vi "main.vi"() -> ()   [LabVIEW 2023] (continued)
20\tFF\tFF\tFF\tFF\tFF\tFF\r\n       952  1FFFFFFF   00000004    8        00\t00\tFF\tFF\tFF\tFF\tFF\tFF\r\n       947  1FFFFFFF   00000004    8        00\t00\tFF\tFF\tFF\tFF\tFF\tFF\r\n       946  18F121F0   00000004    8        09\t16\t00\t00\tFF\tFF\tB0\t01\r\n       993  18F106A7   00000004    8        00\tF7\tFF\tFF\tFF\tFF\tFF\t84\r\n       992  1FFFFFFF   00000004    8        00\t00\tFF\tFF\tFF\tFF\tFF\tFF\r\n       983  0CF102A7   00000004    8        30\t75\tE0\t2E\t80\tFF\tFF\tFD\r\n       983  0CF101A7   00000004    8        68\t00\t97\tCC\t00\t15\t39\t4B\r\n       982  1FFFFFFF   00000004    8        00\t00\tFF\tFF\tFF\tFF\tFF\tFF\r\n       972  1FFFFFFF   00000004    8        00\t00\tFF\tFF\tFF\tFF\tFF\tFF\r\n       963  0CF102A7   00000004    8        30\t75\tE0\t2E\t80\tFF\tFF\tFD\r\n       963  0CF101A7   00000004    8        68\t00\t97\tCC\t00\t15\t39\t4A\r\n       962  1FFFFFFF   00000004    8        00\t20\tFF\tFF\tFF\tFF\tFF\tFF\r\n       952  1FFFFFFF   00000004    8        00\t00\tFF\tFF\tFF\tFF\tFF\tFF\r\n       947  1FFFFFFF   00000004    8        00\t00\tFF\tFF\tFF\tFF\tFF\tFF\r\n      1002  1FFFFFFF   00000004    8        00\t00\tFF\tFF\tFF\tFF\tFF\tFF\r\n       993  18F106A7   00000004    8        00\tF7\tFF\tFF\tFF\tFF\tFF\t84\r\n       992  1FFFFFFF   00000004    8        00\t00\tFF\tFF\tFF\tFF\tFF\tFF\r\n       983  0CF102A7   00000004    8        30\t75\tE0\t2E\t80\tFF\tFF\tFD\r\n       983  0CF101A7   00000004    8        68\t00\t97\tCC\t00\t15\t39\t4B\r\n       982  1FFFFFFF   00000004    8        00\t00\tFF\tFF\tFF\tFF\tFF\tFF\r\n       972  1FFFFFFF   00000004    8        00\t00\tFF\tFF\tFF\tFF\tFF\tFF\r\n       963  0CF102A7   00000004    8        30\t75\tE0\t2E\t80\tFF\tFF\tFD\r\n       963  0CF101A7   00000004    8        68\t00\t97\tCC\t00\t15\t39\t4A\r\n       962  1FFFFFFF   00000004    8        00\t20\tFF\tFF\tFF\tFF\tFF\tFF\r\n       952  1FFFFFFF   00000004    8        00\t00\tFF\tFF\tFF\tFF\tFF\tFF\r\n      1003  0CF101A7   00000004    8        68\t00\t97\tCC\t00\t15\t39\t4C\r\n      1002  1FFFFFFF   00000004    8        00\t00\tFF\tFF\tFF\tFF\tFF\tFF\r\n       993  18F106A7   00000004    8        00\tF7\tFF\tFF\tFF\tFF\tFF\t84\r\n       992  1FFFFFFF   00000004    8        00\t00\tFF\tFF\tFF\tFF\tFF\tFF\r\n       983  0CF102A7   00000004    8        30\t75\tE0\t2E\t80\tFF\tFF\tFD\r\n       983  0CF101A7   00000004    8        68\t00\t97\tCC\t00\t15\t39\t4B\r\n       982  1FFFFFFF   00000004    8        00\t00\tFF\tFF\tFF\tFF\tFF\tFF\r\n       972  1FFFFFFF   00000004    8        00\t00\tFF\tFF\tFF\tFF\tFF\tFF\r\n       963  0CF102A7   00000004    8        30\t75\tE0\t2E\t80\tFF\tFF\tFD\r\n       963  0CF101A7   00000004    8        68\t00\t97\tCC\t00\t15\t39\t4A\r\n       962  1FFFFFFF   00000004    8        00\t20\tFF\tFF\tFF\tFF\tFF\tFF\r\n      1003  0CF102A7   00000004    8        30\t75\tE0\t2E\t80\tFF\tFF\tFD\r\n      1003  0CF101A7   00000004    8        68\t00\t97\tCC\t00\t15\t39\t4C\r\n      1002  1FFFFFFF   00000004    8        00\t00\tFF\tFF\tFF\tFF\tFF\tFF\r\n       993  18F106A7   00000004    8        00\tF7\tFF\tFF\tFF\tFF\tFF\t84\r\n       992  1FFFFFFF   00000004    8        00\t00\tFF\tFF\tFF\tFF\tFF\tFF\r\n       983  0CF102A7   00000004    8        30\t75\tE0\t2E\t80\tFF\tFF\tFD\r\n       983  0CF101A7   00000004    8        68\t00\t97\tCC\t00\t15\t39\t4B\r\n       982  1FFFFFFF   00000004    8        00\t00\tFF\tFF\tFF\tFF\tFF\tFF\r\n       972  1FFFFFFF   00000004    8        00\t00\tFF\tFF\tFF\tFF\tFF\tFF\r\n       963  0CF102A7   00000004    8        30\t75\tE0\t2E\t80\tFF\tFF\tFD\r\n       963  0CF101A7   00000004    8        68\t00\t97\tCC\t00\t15\t39\t4A\r\n      1012  1FFFFFFF   00000004    8        00\t00\tFF\tFF\tFF\tFF\tFF\tFF\r\n      1003  0CF102A7   00000004    8        30\t75\tE0\t2E\t80\tFF\tFF\tFD\r\n      1003  0CF101A7   00000004    8        68\t00\t97\tCC\t00\t15\t39\t4C\r\n      1002  1FFFFFFF   00000004    8        00\t00\tFF\tFF\tFF\tFF\tFF\tFF\r\n       993  18F106A7   00000004    8        00\tF7\tFF\tFF\tFF\tFF\tFF\t84\r\n       992  1FFFFFFF   00000004    8        00\t00\tFF\tFF\tFF\tFF\tFF\tFF\r\n       983  0CF102A7   00000004    8        30\t75\tE0\t2E\t80\tFF\tFF\tFD\r\n       983  0CF101A7   00000004    8        68\t00\t97\tCC\t00\t15\t39\t4B\r\n       982  1FFFFFFF   00000004    8        00\t00\tFF\tFF\tFF\tFF\tFF\tFF\r\n       972  1FFFFFFF   00000004    8        00\t00\tFF\tFF\tFF\tFF\tFF\tFF\r\n       963  0CF102A7   00000004    8        30\t75\tE0\t2E\t80\tFF\tFF\tFD\r\n      1022  1FFFFFFF   00000004    8        00\t20\tFF\tFF\tFF\tFF\tFF\tFF\r\n      1012  1FFFFFFF   00000004    8        00\t00\tFF\tFF\tFF\tFF\tFF\tFF\r\n      1003  0CF102A7   00000004    8        30\t75\tE0\t2E\t80\tFF\tFF\tFD\r\n      1003  0CF101A7   00000004    8        68\t00\t97\tCC\t00\t15\t39\t4C\r\n      1002  1FFFFFFF   00000004    8        00\t00\tFF\tFF\tFF\tFF\tFF\tFF\r\n       993  18F106A7   00000004    8        00\tF7\tFF\tFF\tFF\tFF\tFF\t84\r\n       992  1FFFFFFF   00000004    8        00\t00\tFF\tFF\tFF\tFF\tFF\tFF\r\n       983  0CF102A7   00000004    8        30\t75\tE0\t2E\t80\tFF\tFF\tFD\r\n       983  0CF101A7   00000004    8        68\t00\t97\tCC\t00\t15\t39\t4B\r\n       982  1FFFFFFF   00000004    8        00\t00\tFF\tFF\tFF\tFF\tFF\tFF\r\n       972  1FFFFFFF   00000004    8        00\t00\tFF\tFF\tFF\tFF\tFF\tFF\r\n      1023  0CF101A7   00000004    8        68\t00\t97\tCC\t00\t15\t39\t4D\r\n      1022  1FFFFFFF   00000004    8        00\t20\tFF\tFF\tFF\tFF\tFF\tFF\r\n      1012  1FFFFFFF   00000004    8        00\t00\tFF\tFF\tFF\tFF\tFF\tFF\r\n      1003  0CF102A7   00000004    8        30\t75\tE0\t2E\t80\tFF\tFF\tFD\r\n      1003  0CF101A7   00000004    8        68\t00\t97\tCC\t00\t15\t39\t4C\r\n      1002  1FFFFFFF   00000004    8        00\t00\tFF\tFF\tFF\tFF\tFF\tFF\r\n       993  18F106A7   00000004    8        00\tF7\tFF\tFF\tFF\tFF\tFF\t84\r\n       992  1FFFFFFF   00000004    8        00\t00\tFF\tFF\tFF\tFF\tFF\tFF\r\n       983  0CF102A7   00000004    8        30\t75\tE0\t2E\t80\tFF\tFF\tFD\r\n       983  0CF101A7   00000004    8        68\t00\t97\tCC\t00\t15\t39\t4B\r\n       982  1FFFFFFF   00000004    8        00\t00\tFF\tFF\tFF\tFF\tFF\tFF\r\n      1023  0CF102A7   00000004    8        30\t75\tE0\t2E\t80\tFF\tFF\tFD\r\n      1023  0CF101A7   00000004    8        68\t00\t97\tCC\t00\t15\t39\t4D\r\n      1022  1FFFFFFF   00000004    8        00\t20\tFF\tFF\tFF\tFF\tFF\tFF\r\n      1012  1FFFFFFF   00000004    8        00\t00\tFF\tFF\tFF\tFF\tFF\tFF\r\n      1003  0CF102A7   00000004    8        30\t75\tE0\t2E\t80\tFF\tFF\tFD\r\n      1003  0CF101A7   00000004    8        68\t00\t97\tCC\t00\t15\t39\t4C\r\n      1002  1FFFFFFF   00000004    8        00\t00\tFF\tFF\tFF\tFF\tFF\tFF\r\n       993  18F106A7   00000004    8        00\tF7\tFF\tFF\tFF\tFF\tFF\t84\r\n       992  1FFFFFFF   00000004    8        00\t00\tFF\tFF\tFF\tFF\tFF\tFF\r\n       983  0CF102A7   00000004    8        30\t75\tE0\t2E\t80\tFF\tFF\tFD\r\n       983  0CF101A7   00000004    8        68\t00\t97\tCC\t00\t15\t39\t4B\r\n      1032  1FFFFFFF   00000004    8        00\t00\tFF\tFF\tFF\tFF\tFF\tFF\r\n      1023  0CF102A7   00000004    8        30\t75\tE0\t2E\t80\tFF\tFF\tFD\r\n      1023  0CF101A7   00000004    8        68\t00\t97\tCC\t00\t15\t39\t4D\r\n      1022  1FFFFFFF   00000004    8        00\t20\tFF\tFF\tFF\tFF\tFF\tFF\r\n      1012  1FFFFFFF   00000004    8        00\t00\tFF\tFF\tFF\tFF\tFF\tFF\r\n      1003  0CF102A7   00000004    8        30\t75\tE0\t2E\t80\tFF\tFF\tFD\r\n      1003  0CF101A7   00000004    8        68\t00\t97\tCC\t00\t15\t39\t4C\r\n      1002  1FFFFFFF   00000004    8        00\t00\tFF\tFF\tFF\tFF\tFF\tFF\r\n       993  18F106A7   00000004    8        00\tF7\tFF\tFF\tFF\tFF\tFF\t84\r\n       992  1FFFFFFF   00000004    8        00\t00\tFF\tFF\tFF\tFF\tFF\tFF\r\n       983  0CF102A7   00000004    8        30\t75\tE0\t2E\t80\tFF\tFF\tFD\r\n      1041  18F11FF0   00000004    8        FF\t3F\t90\t68\t88\t1B\t10\t2C\r\n      1032  1FFFFFFF   00000004    8        00\t00\tFF\tFF\tFF\tFF\tFF\tFF\r\n      1023  0CF102A7   00000004    8        30\t75\tE0\t2E\t80\tFF\tFF\tFD\r\n      1023  0CF101A7   00000004    8        68\t00\t97\tCC\t00\t15\t39\t4D\r\n      1022  1FFFFFFF   00000004    8        00\t20\tFF\tFF\tFF\tFF\tFF\tFF\r\n      1012  1FFFFFFF   00000004    8        00\t00\tFF\tFF\tFF\tFF\tFF\tFF\r\n      1003  0CF102A7   00000004    8        30\t75\tE0\t2E\t80\tFF\tFF\tFD\r\n      1003  0CF101A7   00000004    8        68\t00\t97\tCC\t00\t15\t39\t4C\r\n      1002  1FFFFFFF   00000004    8        00\t00\tFF\tFF\tFF\tFF\tFF\tFF\r\n       993  18F106A7   00000004    8        00\tF7\tFF\tFF\tFF\tFF\tFF\t84\r\n       992  1FFFFFFF   00000004    8        00\t00\tFF\tFF\tFF\tFF\tFF\tFF\r\n      1042  18F120F0   00000004    8        2B\t75\t60\tB1\tB0\t01\tFF\tFF\r\n      1041  18F11FF0   00000004    8        FF\t3F\t90\t68\t88\t1B\t10\t2C\r\n      1032  1FFFFFFF   00000004    8        00\t00\tFF\tFF\tFF\tFF\tFF\tFF\r\n      1023  0CF102A7   00000004    8        30\t75\tE0\t2E\t80\tFF\tFF\tFD\r\n      1023  0CF101A7   00000004    8        68\t00\t97\tCC\t00\t15\t39\t4D\r\n      1022  1FFFFFFF   00000004    8        00\t20\tFF\tFF\tFF\tFF\tFF\tFF\r\n      1012  1FFFFFFF   00000004    8        00\t00\tFF\tFF\tFF\tFF\tFF\tFF\r\n      1003  0CF102A7   00000004    8        30\t75\tE0\t2E\t80\tFF\tFF\tFD\r\n      1003  0CF101A7   00000004    8        68\t00\t97\tCC\t00\t15\t39\t4C\r\n      1002  1FFFFFFF   00000004    8        00\t00\tFF\tFF\tFF\tFF\tFF\tFF\r\n       993  18F106A7   00000004    8        00\tF7\tFF\tFF\tFF\tFF\tFF\t84\r\n      1043  0CF101A7   00000004    8        68\t00\t97\tCC\t00\t15\t39\t4E\r\n      1042  18F120F0   00000004    8        2B\t75\t60\tB1\tB0\t01\tFF\tFF\r\n      1041  18F11FF0   00000004    8        FF\t3F\t90\t68\t88\t1B\t10\t2C\r\n      1032  1FFFFFFF   00000004    8        00\t00\tFF\tFF\tFF\tFF\tFF\tFF\r\n      1023  0CF102A7   00000004    8        30\t75\tE0\t2E\t80\tFF\tFF\tFD\r\n      1023  0CF101A7   00000004    8        68\t00\t97\tCC\t00\t15\t39\t4D\r\n      1022  1FFFFFFF   00000004    8        00\t20\tFF\tFF\tFF\tFF\tFF\tFF\r\n      1012  1FFFFFFF   00000004    8        00\t00\tFF\tFF\tFF\tFF\tFF\tFF\r\n      1003  0CF102A7   00000004    8        30\t75\tE0\t2E\t80\tFF\tFF\tFD\r\n      1003  0CF101A7   00000004    8        68\t00\t97\tCC\t00\t15\t39\t4C\r\n      1002  1FFFFFFF   00000004    8        00\t00\tFF\tFF\tFF\tFF\tFF\tFF\r\n      1043  0C3C4D4A   00000004    8        BE\tFF\tFF\t7F\t18\tFF\tFF\t42\r\n      1043  0CF101A7   00000004    8        68\t00\t97\tCC\t00\t15\t39\t4E\r\n      1042  18F120F0   00000004    8        2B\t75\t60\tB1\tB0\t01\tFF\tFF\r\n      1041  18F11FF0   00000004    8        FF\t3F\t90\t68\t88\t1B\t10\t2C\r\n      1032  1FFFFFFF   00000004    8        00\t00\tFF\tFF\tFF\tFF\tFF\tFF\r\n      1023  0CF102A7   00000004    8        30\t75\tE0\t2E\t80\tFF\tFF\tFD\r\n      1023  0CF101A7   00000004    8        68\t00\t97\tCC\t00\t15\t39\t4D\r\n      1022  1FFFFFFF   00000004    8        00\t20\tFF\tFF\tFF\tFF\tFF\tFF\r\n      1012  1FFFFFFF   00000004    8        00\t00\tFF\tFF\tFF\tFF\tFF\tFF\r\n      1003  0CF102A7   00000004    8        30\t75\tE0\t2E\t80\tFF\tFF\tFD\r\n      1003  0CF101A7   00000004    8        68\t00\t97\tCC\t00\t15\t39\t4C\r\n      1044  0CF102A7   00000004    8        30\t75\tE0\t2E\t80\tFF\tFF\tFD\r\n      1043  0C3C4D4A   00000004    8        BE\tFF\tFF\t7F\t18\tFF\tFF\t42\r\n      1043  0CF101A7   00000004    8        68\t00\t97\tCC\t00\t15\t39\t4E\r\n      1042  18F120F0   00000004    8        2B\t75\t60\tB1\tB0\t01\tFF\tFF\r\n      1041  18F11FF0   00000004    8        FF\t3F\t90\t68\t88\t1B\t10\t2C\r\n      1032  1FFFFFFF   00000004    8        00\t00\tFF\tFF\tFF\tFF\tFF\tFF\r\n      1023  0CF102A7   00000004    8        30\t75\tE0\t2E\t80\tFF\tFF\tFD\r\n      1023  0CF101A7   00000004    8        68\t00\t97\tCC\t00\t15\t39\t4D\r\n      1022  1FFFFFFF   00000004    8        00\t20\tFF\tFF\tFF\tFF\tFF\tFF\r\n      1012  1FFFFFFF   00000004    8        00\t00\tFF\tFF\tFF\tFF\tFF\tFF\r\n      1003  0CF102A7   00000004    8        30\t75\tE0\t2E\t80\tFF\tFF\tFD\r\n      1044  0CF103A7   00000004    8        17\t1F\t08\t60\tB1\t1F\t08\t42\r\n      1044  0CF102A7   00000004    8        30\t75\tE0\t2E\t80\tFF\tFF\tFD\r\n      1043  0C3C4D4A   00000004    8        BE\tFF\tFF\t7F\t18\tFF\tFF\t42\r\n      1043  0CF101A7   00000004    8        68\t00\t97\tCC\t00\t15\t39\t4E\r\n      1042  18F120F0   00000004    8        2B\t75\t60\tB1\tB0\t01\tFF\tFF\r\n      1041  18F11FF0   00000004    8        FF\t3F\t90\t68\t88\t1B\t10\t2C\r\n      1032  1FFFFFFF   00000004    8        00\t00\tFF\tFF\tFF\tFF\tFF\tFF\r\n      1023  0CF102A7   00000004    8        30\t75\tE0\t2E\t80\tFF\tFF\tFD\r\n      1023  0CF101A7   00000004    8        68\t00\t97\tCC\t00\t15\t39\t4D\r\n      1022  1FFFFFFF   00000004    8        00\t20\tFF\tFF\tFF\tFF\tFF\tFF\r\n      1012  1FFFFFFF   00000004    8        00\t00\tFF\tFF\tFF\tFF\tFF\tFF\r\n      1045  0CF104A7   00000004    8        F0\t60\t22\tFC\tFF\tFF\tFF\t42\r\n      1044  0CF103A7   00000004    8        17\t1F\t08\t60\tB1\t1F\t08\t42\r\n      1044  0CF102A7   00000004    8        30\t75\tE0\t2E\t80\tFF\tFF\tFD\r\n      1043  0C3C4D4A   00000004    8        BE\tFF\tFF\t7F\t18\tFF\tFF\t42\r\n      1043  0CF101A7   00000004    8        68\t00\t97\tCC\t00\t15\t39\t4E\r\n      1042  18F120F0   00000004    8        2B\t75\t60\tB1\tB0\t01\tFF\tFF\r\n      1041  18F11FF0   00000004    8        FF\t3F\t90\t68\t88\t1B\t10\t2C\r\n      1032  1FFFFFFF   00000004    8        00\t00\tFF\tFF\tFF\tFF\tFF\tFF\r\n      1023  0CF102A7   00000004    8        30\t75\tE0\t2E\t80\tFF\tFF\tFD\r\n      1023  0CF101A7   00000004    8        68\t00\t97\tCC\t00\t15\t39\t4D\r\n      1022  1FFFFFFF   00000004    8        00\t20\tFF\tFF\tFF\tFF\tFF\tFF\r\n      1045  18F106A7   00000004    8        00\tF7\tFF\tFF\tFF\tFF\tFF\t85\r\n      1045  0CF104A7   00000004    8        F0\t60\t22\tFC\tFF\tFF\tFF\t42\r\n      1044  0CF103A7   00000004    8        17\t1F\t08\t60\tB1\t1F\t08\t42\r\n      1044  0CF102A7   00000004    8        30\t75\tE0\t2E\t80\tFF\tFF\tFD\r\n      1043  0C3C4D4A   00000004    8        BE\tFF\tFF\t7F\t18\tFF\tFF\t42\r\n      1043  0CF101A7   00000004    8        68\t00\t97\tCC\t00\t15\t39\t4E\r\n      1042  18F120F0   00000004    8        2B\t75\t60\tB1\tB0\t01\tFF\tFF\r\n      1041  18F11FF0   00000004    8        FF\t3F\t90\t68\t88\t1B\t10\t2C\r\n      1032  1FFFFFFF   00000004    8        00\t00\tFF\tFF\tFF\tFF\tFF\tFF\r\n      1023  0CF102A7   00000004    8        30\t75\tE0\t2E\t80\tFF\tFF\tFD\r\n      1023  0CF101A7   00000004    8        68\t00\t97\tCC\t00\t15\t39\t4D\r\n      1046  18F121F0   00000004    8        09\t18\t00\t00\tFF\tFF\tB0\t01\r\n      1045  18F106A7   00000004    8        00\tF7\tFF\tFF\tFF\tFF\tFF\t85\r\n      1045  0CF104A7   00000004    8        F0\t60\t22\tFC\tFF\tFF\tFF\t42\r\n      1044  0CF103A7   00000004    8        17\t1F\t08\t60\tB1\t1F\t08\t42\r\n      1044  0CF102A7   00000004    8        30\t75\tE0\t2E\t80\tFF\tFF\tFD\r\n      1043  0C3C4D4A   00000004    8        BE\tFF\tFF\t7F\t18\tFF\tFF\t42\r\n      1043  0CF101A7   00000004    8        68\t00\t97\tCC\t00\t15\t39\t4E\r\n      1042  18F120F0   00000004    8        2B\t75\t60\tB1\tB0\t01\tFF\tFF\r\n      1041  18F11FF0   00000004    8        FF\t3F\t90\t68\t88\t1B\t10\t2C\r\n      1032  1FFFFFFF   00000004    8        00\t00\tFF\tFF\tFF\tFF\tFF\tFF\r\n      1023  0CF102A7   00000004    8        30\t75\tE0\t2E\t80\tFF\tFF\tFD\r\n      1047  1FFFFFFF   00000004    8        00\t00\tFF\tFF\tFF\tFF\tFF\tFF\r\n      1046  18F121F0   00000004    8        09\t18\t00\t00\tFF\tFF\tB0\t01\r\n      1045  18F106A7   00000004    8        00\tF7\tFF\tFF\tFF\tFF\tFF\t85\r\n      1045  0CF104A7   00000004    8        F0\t60\t22\tFC\tFF\tFF\tFF\t42\r\n      1044  0CF103A7   00000004    8        17\t1F\t08\t60\tB1\t1F\t08\t42\r\n      1044  0CF102A7   00000004    8        30\t75\tE0\t2E\t80\tFF\tFF\tFD\r\n      1043  0C3C4D4A   00000004    8        BE\tFF\tFF\t7F\t18\tFF\tFF\t42\r\n      1043  0CF101A7   00000004    8        68\t00\t97\tCC\t00\t15\t39\t4E\r\n      1042  18F120F0   00000004    8        2B\t75\t60\tB1\tB0\t01\tFF\tFF\r\n      1041  18F11FF0   00000004    8        FF\t3F\t90\t68\t88\t1B\t10\t2C\r\n      1032  1FFFFFFF   00000004    8        00\t00\tFF\tFF\tFF\tFF\tFF\tFF\r\n      1052  1FFFFFFF   00000004    8        00\t00\tFF\tFF\tFF\tFF\tFF\tFF\r\n      1047  1FFFFFFF   00000004    8        00\t00\tFF\tFF\tFF\tFF\tFF\tFF\r\n      1046  18F121F0   00000004    8        09\t18\t00\t00\tFF\tFF\tB0\t01\r\n      1045  18F106A7   00000004    8        00\tF7\tFF\tFF\tFF\tFF\tFF\t85\r\n      1045  0CF104A7   00000004    8        F0\t60\t22\tFC\tFF\tFF\tFF\t42\r\n      1044  0CF103A7   00000004    8        17\t1F\t08\t60\tB1\t1F\t08\t42\r\n      1044  0CF102A7   00000004    8        30\t75\tE0\t2E\t80\tFF\tFF\tFD\r\n      1043  0C3C4D4A   00000004    8        BE\tFF\tFF\t7F\t18\tFF\tFF\t42\r\n      1043  0CF101A7   00000004    8        68\t00\t97\tCC\t00\t15\t39\t4E\r\n      1042  18F120F0   00000004    8        2B\t75\t60\tB1\tB0\t01\tFF\tFF\r\n      1041  18F11FF0   00000004    8        FF\t3F\t90\t68\t88\t1B\t10\t2C\r\n      1062  1FFFFFFF   00000004    8        00\t20\tFF\tFF\tFF\tFF\tFF\tFF\r\n      1052  1FFFFFFF   00000004    8        00\t00\tFF\tFF\tFF\tFF\tFF\tFF\r\n      1047  1FFFFFFF   00000004    8        00\t00\tFF\tFF\tFF\tFF\tFF\tFF\r\n      1046  18F121F0   00000004    8        09\t18\t00\t00\tFF\tFF\tB0\t01\r\n      1045  18F106A7   00000004    8        00\tF7\tFF\tFF\tFF\tFF\tFF\t85\r\n      1045  0CF104A7   00000004    8        F0\t60\t22\tFC\tFF\tFF\tFF\t42\r\n      1044  0CF103A7   00000004    8        17\t1F\t08\t60\tB1\t1F\t08\t42\r\n      1044  0CF102A7   00000004    8        30\t75\tE0\t2E\t80\tFF\tFF\tFD\r\n      1043  0C3C4D4A   00000004    8        BE\tFF\tFF\t7F\t18\tFF\tFF\t42\r\n      1043  0CF101A7   00000004    8        68\t00\t97\tCC\t00\t15\t39\t4E\r\n      1042  18F120F0   00000004    8        2B\t75\t60\tB1\tB0\t01\tFF\tFF\r\n      1063  0CF101A7   00000004    8        68\t00\t97\tCC\t00\t15\t39\t4F\r\n      1062  1FFFFFFF   00000004    8        00\t20\tFF\tFF\tFF\tFF\tFF\tFF\r\n      1052  1FFFFFFF   00000004    8        00\t00\tFF\tFF\tFF\tFF\tFF\tFF\r\n      1047  1FFFFFFF   00000004    8        00\t00\tFF\tFF\tFF\tFF\tFF\tFF\r\n      1046  18F121F0   00000004    8        09\t18\t00\t00\tFF\tFF\tB0\t01\r\n      1045  18F106A7   00000004    8        00\tF7\tFF\tFF\tFF\tFF\tFF\t85\r\n      1045  0CF104A7   00000004    8        F0\t60\t22\tFC\tFF\tFF\tFF\t42\r\n      1044  0CF103A7   00000004    8        17\t1F\t08\t60\tB1\t1F\t08\t42\r\n      1044  0CF102A7   00000004    8        30\t75\tE0\t2E\t80\tFF\tFF\tFD\r\n      1043  0C3C4D4A   00000004    8        BE\tFF\tFF\t7F\t18\tFF\tFF\t42\r\n      1043  0CF101A7   00000004    8        68\t00\t97\tCC\t00\t15\t39\t4E\r\n      1063  0CF102A7   00000004    8        30\t75\tE0\t2E\t80\tFF\tFF\tFD\r\n      1063  0CF101A7   00000004    8        68\t00\t97\tCC\t00\t15\t39\t4F\r\n      1062  1FFFFFFF   00000004    8        00\t20\tFF\tFF\tFF\tFF\tFF\tFF\r\n      1052  1FFFFFFF   00000004    8        00\t00\tFF\tFF\tFF\tFF\tFF\tFF\r\n      1047  1FFFFFFF   00000004    8        00\t00\tFF\tFF\tFF\tFF\tFF\tFF\r\n      1046  18F121F0   00000004    8        09\t18\t00\t00\tFF\tFF\tB0\t01\r\n      1045  18F106A7   00000004    8        00\tF7\tFF\tFF\tFF\tFF\tFF\t85\r\n      1045  0CF104A7   00000004    8        F0\t60\t22\tFC\tFF\tFF\tFF\t42\r\n      1044  0CF103A7   00000004    8        17\t1F\t08\t60\tB1\t1F\t08\t42\r\n      1044  0CF102A7   00000004    8        30\t75\tE0\t2E\t80\tFF\tFF\tFD\r\n      1043  0C3C4D4A   00000004    8        BE\tFF\tFF\t7F\t18\tFF\tFF\t42\r\n      1072  1FFFFFFF   00000004    8        00\t20\tFF\tFF\tFF\tFF\tFF\tFF\r\n      1063  0CF102A7   00000004    8        30\t75\tE0\t2E\t80\tFF\tFF\tFD\r\n      1063  0CF101A7   00000004    8        68\t00\t97\tCC\t00\t15\t39\t4F\r\n      1062  1FFFFFFF   00000004    8        00\t20\tFF\tFF\tFF\tFF\tFF\tFF\r\n      1052  1FFFFFFF   00000004    8        00\t00\tFF\tFF\tFF\tFF\tFF\tFF\r\n      1047  1FFFFFFF   00000004    8        00\t00\tFF\tFF\tFF\tFF\tFF\tFF\r\n      1046  18F121F0   00000004    8        09\t18\t00\t00\tFF\tFF\tB0\t01\r\n      1045  18F106A7   00000004    8        00\tF7\tFF\tFF\tFF\tFF\tFF\t85\r\n      1045  0CF104A7   00000004    8        F0\t60\t22\tFC\tFF\tFF\tFF\t42\r\n      1044  0CF103A7   00000004    8        17\t1F\t08\t60\tB1\t1F\t08\t42\r\n      1044  0CF102A7   00000004    8        30\t75\tE0\t2E\t80\tFF\tFF\tFD\r\n      1082  1FFFFFFF   00000004    8        00\t20\tFF\tFF\tFF\tFF\tFF\tFF\r\n      1072  1FFFFFFF   00000004    8        00\t20\tFF\tFF\tFF\tFF\tFF\tFF\r\n      1063  0CF102A7   00000004    8        30\t75\tE0\t2E\t80\tFF\tFF\tFD\r\n      1063  0CF101A7   00000004    8        68\t00\t97\tCC\t00\t15\t39\t4F\r\n      1062  1FFFFFFF   00000004    8        00\t20\tFF\tFF\tFF\tFF\tFF\tFF\r\n      1052  1FFFFFFF   00000004    8        00\t00\tFF\tFF\tFF\tFF\tFF\tFF\r\n      1047  1FFFFFFF   00000004    8        00\t00\tFF\tFF\tFF\tFF\tFF\tFF\r\n      1046  18F121F0   00000004    8        09\t18\t00\t00\tFF\tFF\tB0\t01\r\n      1045  18F106A7   00000004    8        00\tF7\tFF\tFF\tFF\tFF\tFF\t85\r\n      1045  0CF104A7   00000004    8        F0\t60\t22\tFC\tFF\tFF\tFF\t42\r\n      1044  0CF103A7   00000004    8        17\t1F\t08\t60\tB1\t1F\t08\t42\r\n      1083  0CF101A7   00000004    8        68\t00\t97\tCC\t00\t15\t39\t50\r\n      1082  1FFFFFFF   00000004    8        00\t20\tFF\tFF\tFF\tFF\tFF\tFF\r\n      1072  1FFFFFFF   00000004    8        00\t20\tFF\tFF\tFF\tFF\tFF\tFF\r\n      1063  0CF102A7   00000004    8        30\t75\tE0\t2E\t80\tFF\tFF\tFD\r\n      1063  0CF101A7   00000004    8        68\t00\t97\tCC\t00\t15\t39\t4F\r\n      1062  1FFFFFFF   00000004    8        00\t20\tFF\tFF\tFF\tFF\tFF\tFF\r\n      1052  1FFFFFFF   00000004    8        00\t00\tFF\tFF\tFF\tFF\tFF\tFF\r\n      1047  1FFFFFFF   00000004    8        00\t00\tFF\tFF\tFF\tFF\tFF\tFF\r\n      1046  18F121F0   00000004    8        09\t18\t00\t00\tFF\tFF\tB0\t01\r\n      1045  18F106A7   00000004    8        00\tF7\tFF\tFF\tFF\tFF\tFF\t85\r\n      1045  0CF104A7   00000004    8        F0\t60\t22\tFC\tFF\tFF\tFF\t42\r\n      1083  0CF102A7   00000004    8        30\t75\tE0\t2E\t80\tFF\tFF\tFD\r\n      1083  0CF101A7   00000004    8        68\t00\t97\tCC\t00\t15\t39\t50\r\n      1082  1FFFFFFF   00000004    8        00\t20\tFF\tFF\tFF\tFF\tFF\tFF\r\n      1072  1FFFFFFF   00000004    8        00\t20\tFF\tFF\tFF\tFF\tFF\tFF\r\n      1063  0CF102A7   00000004    8        30\t75\tE0\t2E\t80\tFF\tFF\tFD\r\n      1063  0CF101A7   00000004    8        68\t00\t97\tCC\t00\t15\t39\t4F\r\n      1062  1FFFFFFF   00000004    8        00\t20\tFF\tFF\tFF\tFF\tFF\tFF\r\n      1052  1FFFFFFF   00000004    8        00\t00\tFF\tFF\tFF\tFF\tFF\tFF\r\n      1047  1FFFFFFF   00000004    8        00\t00\tFF\tFF\tFF\tFF\tFF\tFF\r\n      1046  18F121F0   00000004    8        09\t18\t00\t00\tFF\tFF\tB0\t01\r\n      1045  18F106A7   00000004    8        00\tF7\tFF\tFF\tFF\tFF\tFF\t85\r\n      1092  1FFFFFFF   00000004    8        00\t00\tFF\tFF\tFF\tFF\tFF\tFF\r\n      1083  0CF102A7   00000004    8        30\t75\tE0\t2E\t80\tFF\tFF\tFD\r\n      1083  0CF101A7   00000004    8        68\t00\t97\tCC\t00\t15\t39\t50\r\n      1082  1FFFFFFF   00000004    8        00\t20\tFF\tFF\tFF\tFF\tFF\tFF\r\n      1072  1FFFFFFF   00000004    8        00\t20\tFF\tFF\tFF\tFF\tFF\tFF\r\n      1063  0CF102A7   00000004    8        30\t75\tE0\t2E\t80\tFF\tFF\tFD\r\n      1063  0CF101A7   00000004    8        68\t00\t97\tCC\t00\t15\t39\t4F\r\n      1062  1FFFFFFF   00000004    8        00\t20\tFF\tFF\tFF\tFF\tFF\tFF\r\n      1052  1FFFFFFF   00000004    8        00\t00\tFF\tFF\tFF\tFF\tFF\tFF\r\n      1047  1FFFFFFF   00000004    8        00\t00\tFF\tFF\tFF\tFF\tFF\tFF\r\n      1046  18F121F0   00000004    8        09\t18\t00\t00\tFF\tFF\tB0\t01\r\n      1093  18F106A7   00000004    8        00\tF7\tFF\tFF\tFF\tFF\tFF\t86\r\n      1092  1FFFFFFF   00000004    8        00\t00\tFF\tFF\tFF\tFF\tFF\tFF\r\n      1083  0CF102A7   00000004    8        30\t75\tE0\t2E\t80\tFF\tFF\tFD\r\n      1083  0CF101A7   00000004    8        68\t00\t97\tCC\t00\t15\t39\t50\r\n      1082  1FFFFFFF   00000004    8        00\t20\tFF\tFF\tFF\tFF\tFF\tFF\r\n      1072  1FFFFFFF   00000004    8        00\t20\tFF\tFF\tFF\tFF\tFF\tFF\r\n      1063  0CF102A7   00000004    8        30\t75\tE0\t2E\t80\tFF\tFF\tFD\r\n      1063  0CF101A7   00000004    8        68\t00\t97\tCC\t00\t15\t39\t4F\r\n      1062  1FFFFFFF   00000004    8        00\t20\tFF\tFF\tFF\tFF\tFF\tFF\r\n      1052  1FFFFFFF   00000004    8        00\t00\tFF\tFF\tFF\tFF\tFF\tFF\r\n      1047  1FFFFFFF   00000004    8        00\t00\tFF\tFF\tFF\tFF\tFF\tFF\r\n      1102  1FFFFFFF   00000004    8        00\t20\tFF\tFF\tFF\tFF\tFF\tFF\r\n      1093  18F106A7   00000004    8        00\tF7\tFF\tFF\tFF\tFF\tFF\t86\r\n      1092  1FFFFFFF   00000004    8        00\t00\tFF\tFF\tFF\tFF\tFF\tFF\r\n      1083  0CF102A7   00000004    8        30\t75\tE0\t2E\t80\tFF\tFF\tFD\r\n      1083  0CF101A7   00000004    8        68\t00\t97\tCC\t00\t15\t39\t50\r\n      1082  1FFFFFFF   00000004    8        00\t20\tFF\tFF\tFF\tFF\tFF\tFF\r\n      1072  1FFFFFFF   00000004    8        00\t20\tFF\tFF\tFF\tFF\tFF\tFF\r\n      1063  0CF102A7   00000004    8        30\t75\tE0\t2E\t80\tFF\tFF\tFD\r\n      1063  0CF101A7   00000004    8        68\t00\t97\tCC\t00\t15\t39\t4F\r\n      1062  1FFFFFFF   00000004    8        00\t20\tFF\tFF\tFF\tFF\tFF\tFF\r\n      1052  1FFFFFFF   00000004    8        00\t00\tFF\tFF\tFF\tFF\tFF\tFF\r\n      1103  0CF101A7   00000004    8        68\t00\t97\tCC\t00\t15\t39\t51\r\n      1102  1FFFFFFF   00000004    8        00\t20\tFF\tFF\tFF\tFF\tFF\tFF\r\n      1093  18F106A7   00000004    8        00\tF7\tFF\tFF\tFF\tFF\tFF\t86\r\n      1092  1FFFFFFF   00000004    8        00\t00\tFF\tFF\tFF\tFF\tFF\tFF\r\n      1083  0CF102A7   00000004    8        30\t75\tE0\t2E\t80\tFF\tFF\tFD\r\n      1083  0CF101A7   00000004    8        68\t00\t97\tCC\t00\t15\t39\t50\r\n      1082  1FFFFFFF   00000004    8        00\t20\tFF\tFF\tFF\tFF\tFF\tFF\r\n      1072  1FFFFFFF   00000004    8        00\t20\tFF\tFF\tFF\tFF\tFF\tFF\r\n      1063  0CF102A7   00000004    8        30\t75\tE0\t2E\t80\tFF\tFF\tFD\r\n      1063  0CF101A7   00000004    8        68\t00\t97\tCC\t00\t15\t39\t4F\r\n      1062  1FFFFFFF   00000004    8        00\t20\tFF\tFF\tFF\tFF\tFF\tFF\r\n      1103  0CF102A7   00000004    8        30\t75\tE0\t2E\t80\tFF\tFF\tFD\r\n      1103  0CF101A7   00000004    8        68\t00\t97\tCC\t00\t15\t39\t51\r\n      1102  1FFFFFFF   00000004    8        00\t20\tFF\tFF\tFF\tFF\tFF\tFF\r\n      1093  18F106A7   00000004    8        00\tF7\tFF\tFF\tFF\tFF\tFF\t86\r\n      1092  1FFFFFFF   00000004    8        00\t00\tFF\tFF\tFF\tFF\tFF\tFF\r\n      1083  0CF102A7   00000004    8        30\t75\tE0\t2E\t80\tFF\tFF\tFD\r\n      1083  0CF101A7   00000004    8        68\t00\t97\tCC\t00\t15\t39\t50\r\n      1082  1FFFFFFF   00000004    8        00\t20\tFF\tFF\tFF\tFF\tFF\tFF\r\n      1072  1FFFFFFF   00000004    8        00\t20\tFF\tFF\tFF\tFF\tFF\tFF\r\n      1063  0CF102A7   00000004    8        30\t75\tE0\t2E\t80\tFF\tFF\tFD\r\n      1063  0CF101A7   00000004    8        68\t00\t97\tCC\t00\t15\t39\t4F\r\n      1112  1FFFFFFF   00000004    8        00\t20\tFF\tFF\tFF\tFF\tFF\tFF\r\n      1103  0CF102A7   00000004    8        30\t75\tE0\t2E\t80\tFF\tFF\tFD\r\n      1103  0CF101A7   00000004    8        68\t00\t97\tCC\t00\t15\t39\t51\r\n      1102  1FFFFFFF   00000004    8        00\t20\tFF\tFF\tFF\tFF\tFF\tFF\r\n      1093  18F106A7   00000004    8        00\tF7\tFF\tFF\tFF\tFF\tFF\t86\r\n      1092  1FFFFFFF   00000004    8        00\t00\tFF\tFF\tFF\tFF\tFF\tFF\r\n      1083  0CF102A7   00000004    8        30\t75\tE0\t2E\t80\tFF\tFF\tFD\r\n      1083  0CF101A7   00000004    8        68\t00\t97\tCC\t00\t15\t39\t50\r\n      1082  1FFFFFFF   00000004    8        00\t20\tFF\tFF\tFF\tFF\tFF\tFF\r\n      1072  1FFFFFFF   00000004    8        00\t20\tFF\tFF\tFF\tFF\tFF\tFF\r\n      1063  0CF102A7   00000004    8        30\t75\tE0\t2E\t80\tFF\tFF\tFD\r\n      1122  1FFFFFFF   00000004    8        00\t20\tFF\tFF\tFF\tFF\tFF\tFF\r\n      1112  1FFFFFFF   00000004    8        00\t20\tFF\tFF\tFF\tFF\tFF\tFF\r\n      1103  0CF102A7   00000004    8        30\t75\tE0\t2E\t80\tFF\tFF\tFD\r\n      1103  0CF101A7   00000004    8        68\t00\t97\tCC\t00\t15\t39\t51\r\n      1102  1FFFFFFF   00000004    8        00\t20\tFF\tFF\tFF\tFF\tFF\tFF\r\n      1093  18F106A7   00000004    8        00\tF7\tFF\tFF\tFF\tFF\tFF\t86\r\n      1092  1FFFFFFF   00000004    8        00\t00\tFF\tFF\tFF\tFF\tFF\tFF\r\n      1083  0CF102A7   00000004    8        30\t75\tE0\t2E\t80\tFF\tFF\tFD\r\n      1083  0CF101A7   00000004    8        68\t00\t97\tCC\t00\t15\t39\t50\r\n      1082  1FFFFFFF   00000004    8        00\t20\tFF\tFF\tFF\tFF\tFF\tFF\r\n      1072  1FFFFFFF   00000004    8        00\t20\tFF\tFF\tFF\tFF\tFF\tFF\r\n      1123  0CF101A7   00000004    8        68\t00\t97\tCC\t00\t15\t39\t52\r\n      1122  1FFFFFFF   00000004    8        00\t20\tFF\tFF\tFF\tFF\tFF\tFF\r\n      1112  1FFFFFFF   00000004    8        00\t20\tFF\tFF\tFF\tFF\tFF\tFF\r\n      1103  0CF102A7   00000004    8        30\t75\tE0\t2E\t80\tFF\tFF\tFD\r\n      1103  0CF101A7   00000004    8        68\t00\t97\tCC\t00\t15\t39\t51\r\n      1102  1FFFFFFF   00000004    8        00\t20\tFF\tFF\tFF\tFF\tFF\tFF\r\n      1093  18F106A7   00000004    8        00\tF7\tFF\tFF\tFF\tFF\tFF\t86\r\n      1092  1FFFFFFF   00000004    8        00\t00\tFF\tFF\tFF\tFF\tFF\tFF\r\n      1083  0CF102A7   00000004    8        30\t75\tE0\t2E\t80\tFF\tFF\tFD\r\n      1083  0CF101A7   00000004    8        68\t00\t97\tCC\t00\t15\t39\t50\r\n      1082  1FFFFFFF   00000004    8        00\t20\tFF\tFF\tFF\tFF\tFF\tFF\r\n      1123  0CF102A7   00000004    8        30\t75\tE0\t2E\t80\tFF\tFF\tFD\r\n      1123  0CF101A7   00000004    8        68\t00\t97\tCC\t00\t15\t39\t52\r\n      1122  1FFFFFFF   00000004    8        00\t20\tFF\tFF\tFF\tFF\tFF\tFF\r\n      1112  1FFFFFFF   00000004    8        00\t20\tFF\tFF\tFF\tFF\tFF\tFF\r\n      1103  0CF102A7   00000004    8        30\t75\tE0\t2E\t80\tFF\tFF\tFD\r\n      1103  0CF101A7   00000004    8        68\t00\t97\tCC\t00\t15\t39\t51\r\n      1102  1FFFFFFF   00000004    8        00\t20\tFF\tFF\tFF\tFF\tFF\tFF\r\n      1093  18F106A7   00000004    8        00\tF7\tFF\tFF\tFF\tFF\tFF\t86\r\n      1092  1FFFFFFF   00000004    8        00\t00\tFF\tFF\tFF\tFF\tFF\tFF\r\n      1083  0CF102A7   00000004    8        30\t75\tE0\t2E\t80\tFF\tFF\tFD\r\n      1083  0CF101A7   00000004    8        68\t00\t97\tCC\t00\t15\t39\t50\r\n      1132  1FFFFFFF   00000004    8        00\t20\tFF\tFF\tFF\tFF\tFF\tFF\r\n      1123  0CF102A7   00000004    8        30\t75\tE0\t2E\t80\tFF\tFF\tFD\r\n      1123  0CF101A7   00000004    8        68\t00\t97\tCC\t00\t15\t39\t52\r\n      1122  1FFFFFFF   00000004    8        00\t20\tFF\tFF\tFF\tFF\tFF\tFF\r\n      1112  1FFFFFFF   00000004    8        00\t20\tFF\tFF\tFF\tFF\tFF\tFF\r\n      1103  0CF102A7   00000004    8        30\t75\tE0\t2E\t80\tFF\tFF\tFD\r\n      1103  0CF101A7   00000004    8        68\t00\t97\tCC\t00\t15\t39\t51\r\n      1102  1FFFFFFF   00000004    8        00\t20\tFF\tFF\tFF\tFF\tFF\tFF\r\n      1093  18F106A7   00000004    8        00\tF7\tFF\tFF\tFF\tFF\tFF\t86\r\n      1092  1FFFFFFF   00000004    8        00\t00\tFF\tFF\tFF\tFF\tFF\tFF\r\n      1083  0CF102A7   00000004    8        30\t75\tE0\t2E\t80\tFF\tFF\tFD\r\n      1141  18F11FF0   00000004    8        FF\t3F\t90\t68\t88\t1B\t10\t3C\r\n      1132  1FFFFFFF   00000004    8        00\t20\tFF\tFF\tFF\tFF\tFF\tFF\r\n      1123  0CF102A7   00000004    8        30\t75\tE0\t2E\t80\tFF\tFF\tFD\r\n      1123  0CF101A7   00000004    8        68\t00\t97\tCC\t00\t15\t39\t52\r\n      1122  1FFFFFFF   00000004    8        00\t20\tFF\tFF\tFF\tFF\tFF\tFF\r\n      1112  1FFFFFFF   00000004    8        00\t20\tFF\tFF\tFF\tFF\tFF\tFF\r\n      1103  0CF102A7   00000004    8        30\t75\tE0\t2E\t80\tFF\tFF\tFD\r\n      1103  0CF101A7   00000004    8        68\t00\t97\tCC\t00\t15\t39\t51\r\n      1102  1FFFFFFF   00000004    8        00\t20\tFF\tFF\tFF\tFF\tFF\tFF\r\n      1093  18F106A7   00000004    8        00\tF7\tFF\tFF\tFF\tFF\tFF\t86\r\n      1092  1FFFFFFF   00000004    8        00\t00\tFF\tFF\tFF\tFF\tFF\tFF\r\n      1142  18F120F0   00000004    8        2B\t75\t60\tB1\tB0\t01\tFF\tFF\r\n      1141  18F11FF0   00000004    8        FF\t3F\t90\t68\t88\t1B\t10\t3C\r\n      1132  1FFFFFFF   00000004    8        00\t20\tFF\tFF\tFF\tFF\tFF\tFF\r\n      1123  0CF102A7   00000004    8        30\t75\tE0\t2E\t80\tFF\tFF\tFD\r\n      1123  0CF101A7   00000004    8        68\t00\t97\tCC\t00\t15\t39\t52\r\n      1122  1FFFFFFF   00000004    8        00\t20\tFF\tFF\tFF\tFF\tFF\tFF\r\n      1112  1FFFFFFF   00000004    8        00\t20\tFF\tFF\tFF\tFF\tFF\tFF\r\n      1103  0CF102A7   00000004    8        30\t75\tE0\t2E\t80\tFF\tFF\tFD\r\n      1103  0CF101A7   00000004    8        68\t00\t97\tCC\t00\t15\t39\t51\r\n      1102  1FFFFFFF   00000004    8        00\t20\tFF\tFF\tFF\tFF\tFF\tFF\r\n      1093  18F106A7   00000004    8        00\tF7\tFF\tFF\tFF\tFF\tFF\t86\r\n      1143  0CF101A7   00000004    8        68\t00\t97\tCC\t00\t15\t39\t53\r\n      1142  18F120F0   00000004    8        2B\t75\t60\tB1\tB0\t01\tFF\tFF\r\n      1141  18F11FF0   00000004    8        FF\t3F\t90\t68\t88\t1B\t10\t3C\r\n      1132  1FFFFFFF   00000004    8        00\t20\tFF\tFF\tFF\tFF\tFF\tFF\r\n      1123  0CF102A7   00000004    8        30\t75\tE0\t2E\t80\tFF\tFF\tFD\r\n      1123  0CF101A7   00000004    8        68\t00\t97\tCC\t00\t15\t39\t52\r\n      1122  1FFFFFFF   00000004    8        00\t20\tFF\tFF\tFF\tFF\tFF\tFF\r\n      1112  1FFFFFFF   00000004    8        00\t20\tFF\tFF\tFF\tFF\tFF\tFF\r\n      1103  0CF102A7   00000004    8        30\t75\tE0\t2E\t80\tFF\tFF\tFD\r\n      1103  0CF101A7   00000004    8        68\t00\t97\tCC\t00\t15\t39\t51\r\n      1102  1FFFFFFF   00000004    8        00\t20\tFF\tFF\tFF\tFF\tFF\tFF\r\n      1143  0C3C4D4A   00000004    8        BE\tFF\tFF\t7F\t18\tFF\tFF\t43\r\n      1143  0CF101A7   00000004    8        68\t00\t97\tCC\t00\t15\t39\t53\r\n      1142  18F120F0   00000004    8        2B\t75\t60\tB1\tB0\t01\tFF\tFF\r\n      1141  18F11FF0   00000004    8        FF\t3F\t90\t68\t88\t1B\t10\t3C\r\n      1132  1FFFFFFF   00000004    8        00\t20\tFF\tFF\tFF\tFF\tFF\tFF\r\n      1123  0CF102A7   00000004    8        30\t75\tE0\t2E\t80\tFF\tFF\tFD\r\n      1123  0CF101A7   00000004    8        68\t00\t97\tCC\t00\t15\t39\t52\r\n      1122  1FFFFFFF   00000004    8        00\t20\tFF\tFF\tFF\tFF\tFF\tFF\r\n      1112  1FFFFFFF   00000004    8        00\t20\tFF\tFF\tFF\tFF\tFF\tFF\r\n      1103  0CF102A7   00000004    8        30\t75\tE0\t2E\t80\tFF\tFF\tFD\r\n      1103  0CF101A7   00000004    8        68\t00\t97\tCC\t00\t15\t39\t51\r\n      1144  0CF102A7   00000004    8        30\t75\tE0\t2E\t80\tFF\tFF\tFD\r\n      1143  0C3C4D4A   00000004    8        BE\tFF\tFF\t7F\t18\tFF\tFF\t43\r\n      1143  0CF101A7   00000004    8        68\t00\t97\tCC\t00\t15\t39\t53\r\n      1142  18F120F0   00000004    8        2B\t75\t60\tB1\tB0\t01\tFF\tFF\r\n      1141  18F11FF0   00000004    8        FF\t3F\t90\t68\t88\t1B\t10\t3C\r\n      1132  1FFFFFFF   00000004    8        00\t20\tFF\tFF\tFF\tFF\tFF\tFF\r\n      1123  0CF102A7   00000004    8        30\t75\tE0\t2E\t80\tFF\tFF\tFD\r\n      1123  0CF101A7   00000004    8        68\t00\t97\tCC\t00\t15\t39\t52\r\n      1122  1FFFFFFF   00000004    8        00\t20\tFF\tFF\tFF\tFF\tFF\tFF\r\n      1112  1FFFFFFF   00000004    8        00\t20\tFF\tFF\tFF\tFF\tFF\tFF\r\n      1103  0CF102A7   00000004    8        30\t75\tE0\t2E\t80\tFF\tFF\tFD\r\n      1144  0CF103A7   00000004    8        17\t1F\t08\t60\tB1\t1F\t08\t43\r\n      1144  0CF102A7   00000004    8        30\t75\tE0\t2E\t80\tFF\tFF\tFD\r\n      1143  0C3C4D4A   00000004    8        BE\tFF\tFF\t7F\t18\tFF\tFF\t43\r\n      1143  0CF101A7   00000004    8        68\t00\t97\tCC\t00\t15\t39\t53\r\n      1142  18F120F0   00000004    8        2B\t75\t60\tB1\tB0\t01\tFF\tFF\r\n      1141  18F11FF0   00000004    8        FF\t3F\t90\t68\t88\t1B\t10\t3C\r\n      1132  1FFFFFFF   00000004    8        00\t20\tFF\tFF\tFF\tFF\tFF\tFF\r\n      1123  0CF102A7   00000004    8        30\t75\tE0\t2E\t80\tFF\tFF\tFD\r\n      1123  0CF101A7   00000004    8        68\t00\t97\tCC\t00\t15\t39\t52\r\n      1122  1FFFFFFF   00000004    8        00\t20\tFF\tFF\tFF\tFF\tFF\tFF\r\n      1112  1FFFFFFF   00000004    8        00\t20\tFF\tFF\tFF\tFF\tFF\tFF\r\n      1145  0CF104A7   00000004    8        F0\t60\t22\tFC\tFF\tFF\tFF\t43\r\n      1144  0CF103A7   00000004    8        17\t1F\t08\t60\tB1\t1F\t08\t43\r\n      1144  0CF102A7   00000004    8        30\t75\tE0\t2E\t80\tFF\tFF\tFD\r\n      1143  0C3C4D4A   00000004    8        BE\tFF\tFF\t7F\t18\tFF\tFF\t43\r\n      1143  0CF101A7   00000004    8        68\t00\t97\tCC\t00\t15\t39\t53\r\n      1142  18F120F0   00000004    8        2B\t75\t60\tB1\tB0\t01\tFF\tFF\r\n      1141  18F11FF0   00000004    8        FF\t3F\t90\t68\t88\t1B\t10\t3C\r\n      1132  1FFFFFFF   00000004    8        00\t20\tFF\tFF\tFF\tFF\tFF\tFF\r\n      1123  0CF102A7   00000004    8        30\t75\tE0\t2E\t80\tFF\tFF\tFD\r\n      1123  0CF101A7   00000004    8        68\t00\t97\tCC\t00\t15\t39\t52\r\n      1122  1FFFFFFF   00000004    8        00\t20\tFF\tFF\tFF\tFF\tFF\tFF\r\n      1145  18F106A7   00000004    8        00\tF7\tFF\tFF\tFF\tFF\tFF\t87\r\n      1145  0CF104A7   00000004    8        F0\t60\t22\tFC\tFF\tFF\tFF\t43\r\n      1144  0CF103A7   00000004    8        17\t1F\t08\t60\tB1\t1F\t08\t43\r\n      1144  0CF102A7   00000004    8        30\t75\tE0\t2E\t80\tFF\tFF\tFD\r\n      1143  0C3C4D4A   00000004    8        BE\tFF\tFF\t7F\t18\tFF\tFF\t43\r\n      1143  0CF101A7   00000004    8        68\t00\t97\tCC\t00\t15\t39\t53\r\n      1142  18F120F0   00000004    8        2B\t75\t60\tB1\tB0\t01\tFF\tFF\r\n      1141  18F11FF0   00000004    8        FF\t3F\t90\t68\t88\t1B\t10\t3C\r\n      1132  1FFFFFFF   00000004    8        00\t20\tFF\tFF\tFF\tFF\tFF\tFF\r\n      1123  0CF102A7   00000004    8        30\t75\tE0\t2E\t80\tFF\tFF\tFD\r\n      1123  0CF101A7   00000004    8        68\t00\t97\tCC\t00\t15\t39\t52\r\n      1146  18F108A7   00000004    8        F0\t00\t00\tFF\tFF\tFF\tFF\t40\r\n      1145  18F106A7   00000004    8        00\tF7\tFF\tFF\tFF\tFF\tFF\t87\r\n      1145  0CF104A7   00000004    8        F0\t60\t22\tFC\tFF\tFF\tFF\t43\r\n      1144  0CF103A7   00000004    8        17\t1F\t08\t60\tB1\t1F\t08\t43\r\n      1144  0CF102A7   00000004    8        30\t75\tE0\t2E\t80\tFF\tFF\tFD\r\n      1143  0C3C4D4A   00000004    8        BE\tFF\tFF\t7F\t18\tFF\tFF\t43\r\n      1143  0CF101A7   00000004    8        68\t00\t97\tCC\t00\t15\t39\t53\r\n      1142  18F120F0   00000004    8        2B\t75\t60\tB1\tB0\t01\tFF\tFF\r\n      1141  18F11FF0   00000004    8        FF\t3F\t90\t68\t88\t1B\t10\t3C\r\n      1132  1FFFFFFF   00000004    8        00\t20\tFF\tFF\tFF\tFF\tFF\tFF\r\n      1123  0CF102A7   00000004    8        30\t75\tE0\t2E\t80\tFF\tFF\tFD\r\n      1147  18F121F0   00000004    8        09\t18\t00\t00\tFF\tFF\tB0\t01\r\n      1146  18F108A7   00000004    8        F0\t00\t00\tFF\tFF\tFF\tFF\t40\r\n      1145  18F106A7   00000004    8        00\tF7\tFF\tFF\tFF\tFF\tFF\t87\r\n      1145  0CF104A7   00000004  
